vi "Initialize_Control.vi"(0 "ERD Loop":refnum<queue>, 2 "GEA2":refnum<queue>, 7 "Receive Loop":refnum<user-event>, 9 "UI Loop Error":refnum<user-event>, 11 "Error In":errorcluster) -> (15 "Error Out":errorcluster)   [LabVIEW 2023]
uses:
  type defs/ERD_Data_Loop_Control.ctl
  type defs/ERD_Loop_States.ctl
  GExplorer Support/typedefs/GExplorer_Data_Cluster.ctl
  type defs/DAQ_States.ctl
  type defs/Error_Command.ctl
  type defs/ERD_Loop_Control_Command.ctl
  type defs/GEA2_Control_Command.ctl
  type defs/DAQ_Control.ctl
panel:
  in  "DAQ Queue":refnum<queue>
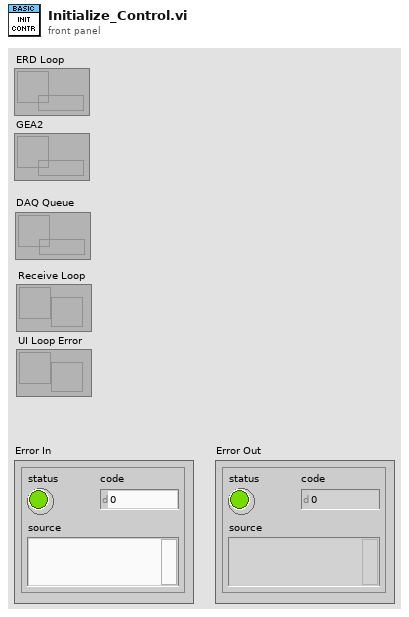
[diagram p1: front panel]
types:
  T1 = typedef "DAQ_Control.ctl" = enum16{"Initialize", "Shutdown", "Exit"}
  T2 = typedef "GEA2_Control_Command.ctl" = enum16{"Initialize", "Shutdown"}
  T3 = typedef "ERD_Loop_Control_Command.ctl" = enum16{"Initialize", "Shutdown"}
  T4 = typedef "Error_Command.ctl" = enum16{"Initialize", "Handle Errors", "Report Errors"}
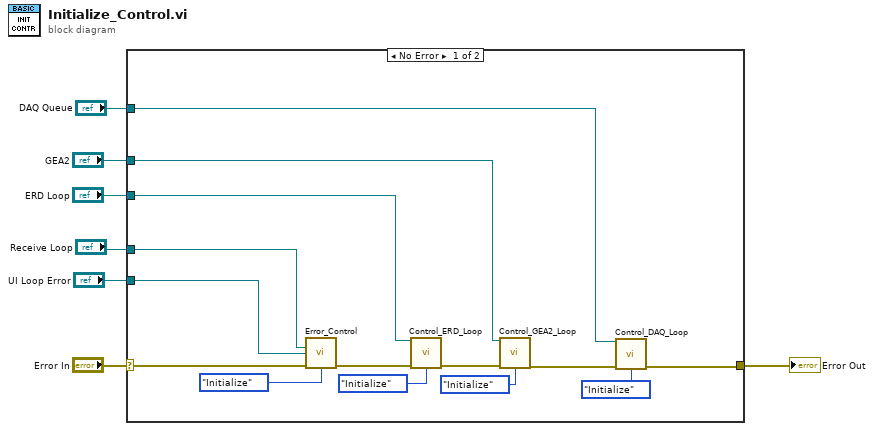
[diagram p0: block diagram]
diagram:
  n1 = case shown="No Error" "Error In" {
    selector: "Error In" -> [w16 w22]
    tunnel: [w10 w22] -> w6
    tunnel: "Receive Loop" -> [w12 _]
    tunnel: "ERD Loop" -> [w15 _]
    tunnel: "GEA2" -> [w14 _]
    tunnel: "UI Loop Error" -> [w13 _]
    tunnel: "DAQ Queue" -> [w8 _]
    frame No Error {
      n2 = call "Error_Control.vi"("Command (Handle Errors)"=Error_Command."Initialize", "Receive Loop"=w12, "UI Loop Error"=w13, "Error In"=w16) -> ("Error Out"=w17:errorcluster)  [unwired: 11 in]
      n3 = call "Control_ERD_Loop.vi"("ERD Loop"=w15, "Command (ERD Loop Control)"=ERD_Loop_Control_Command."Initialize", "Error In"=w17) -> ("Error Out"=w19:errorcluster)  [unwired: 12 in]
      n4 = call "Control_GEA2_Loop.vi"("GEA2"=w14, "Command (ERD Loop Control)"=GEA2_Control_Command."Initialize", "Error In"=w19) -> ("Error Out"=w11:errorcluster)  [unwired: 12 in]
      n5 = call "Control_DAQ_Loop.vi"("DAQ"=w8, "DAQ Control"=DAQ_Control."Initialize", "Error In"=w11) -> ("Error Out"=w10:errorcluster)  [unwired: 12 in]
    }
    frame Error {
    }
  }
  "Error Out" <- w6
